vi "3.2.vi"() -> ()   [LabVIEW 2020]
panel:
  out "min S2":dbl
  out "max S2":dbl
  out "max S1":dbl
  out "min S1":dbl
  out "Grafica":cluster{dbl, dbl}[](graph)
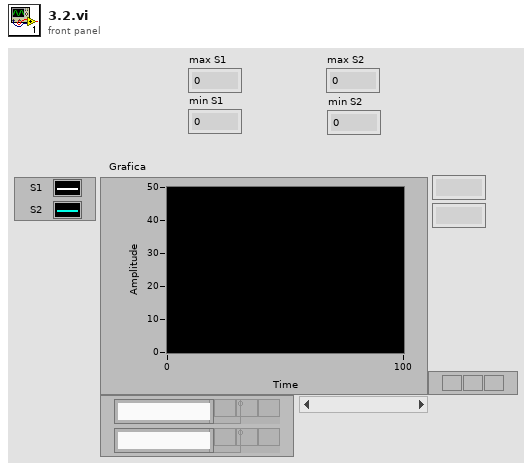
[diagram p1: front panel]
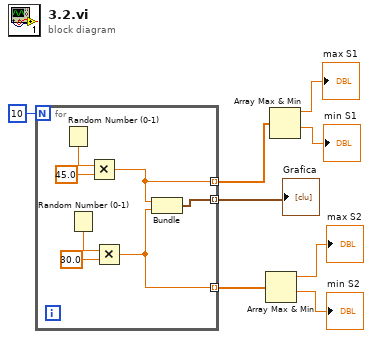
[diagram p0: block diagram]
diagram:
  n1 = for {
    N: 10 -> [_]
    tunnel: [w11] -> w7 mode=indexing
    tunnel: [w10] -> w6 mode=indexing
    tunnel: [w9] -> w3 mode=indexing
    n2 = Random Number (0-1)() -> (number: 0 to 1=w15:dbl)
    n3 = Random Number (0-1)() -> (number: 0 to 1=w13:dbl)
    n4 = Multiply(x=w15, y=45.0) -> (x*y=w10:dbl)
    n5 = Multiply(x=w13, y=30.0) -> (x*y=w9:dbl)
    n6 = Bundle(w10, w9) -> (w11:cluster{dbl, dbl})  [unwired: 1 in]
  }
  "Grafica" <- w7
  n7 = Array Max & Min(array=w3) -> (max value=→"max S2":dbl, min value=→"min S2":dbl)  [unwired: 2 out]
  n8 = Array Max & Min(array=w6) -> (max value=→"max S1":dbl, min value=→"min S1":dbl)  [unwired: 2 out]
